vi "ResetAndDefineConstants.vi"   [LabVIEW 2020]
doc: "This VI sets constants and resets the global variables."
uses:
  constants.vi
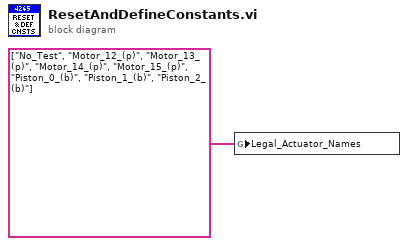
[diagram p0: block diagram]
diagram:
  n1 = global write "constants.vi" "Legal_Actuator_Names"(string[] ["No_Test", "Motor_12_(p)", "Motor_13_(p)", "Motor_14_(p)", "Motor_15_(p)", "Piston_0_(b)", "Piston_1_(b)", "Piston_2_(b)"] ("appended array")) -> ()
